vi "Terminal-Global-SetValues.vi"() -> ()   [LabVIEW 2014]
panel:
  out "载荷谱行索引":dbl
  in  "载荷谱已执行轮次":u32
  in  "载荷谱执行总轮次":u32
  in  "试验日期":string
  out "载荷谱":string[][](table)
  in  "轴承类型":string
  in  "试验人员姓名":string
  in  "试验名称":string
  in  "供油流量":u16
  in  "供油油温":u16
  in  "径向载荷":u16
  in  "轴向载荷":u16
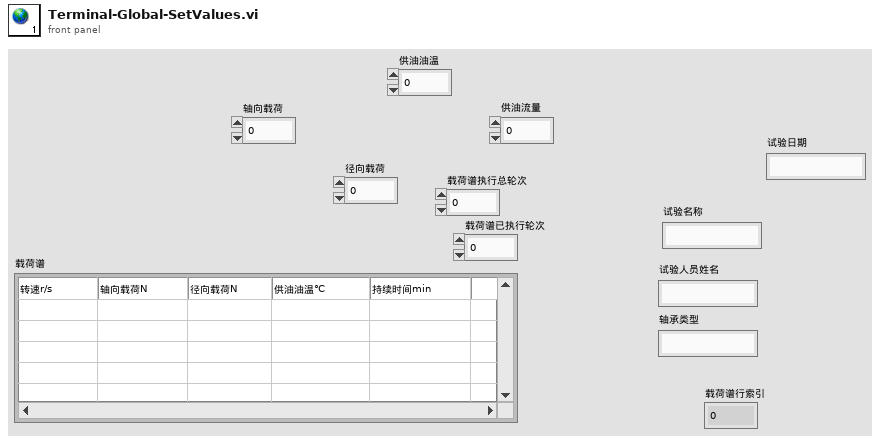
[diagram p1: front panel]
diagram:
